vi "Send Core.vi"(6 "Severity Code (info)":T1=enum."info", 8 "Error In":errorcluster, 9 "Message Content":string, 10 "Message Tag":string, 11 "CS++DSCMsgLogger in":refnum<class "CS++DSCMsgLogger.lvclass">) -> (0 "Error Out":errorcluster, 3 "CS++DSCMsgLogger out":refnum<class "CS++DSCMsgLogger.lvclass">)   [LabVIEW 2014, in "CS++DSCMsgLogger.lvlib" / "CS++DSCMsgLogger.lvclass"]
doc: "Send mesage to central message logger."
uses:
  CS++DSCMsgLogger.lvclass
  CSPP_Core/Libraries/Base/Severity.ctl
  CS++DSCMsgLogger.lvclass/CS++DSCMsgLogger.ctl
  <vilib>/Utility/error.llb/DialogType.ctl
  CSPP_Core/Libraries/Base/CS++Base.lvlib
  <vilib>/lvdsc/NI_DSC.lvlib
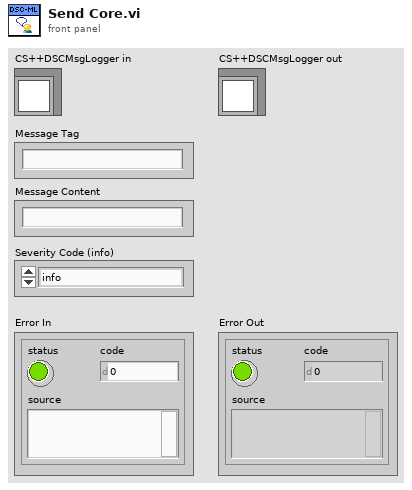
[diagram p1: front panel]
types:
  T1 = typedef "CS++Base.lvlib/Severity.ctl" = enum16{"emergency", "alert", "critical", "error", "warning", "notice", "info", "debug"}
  T2 = typedef "DialogType.ctl" = u16
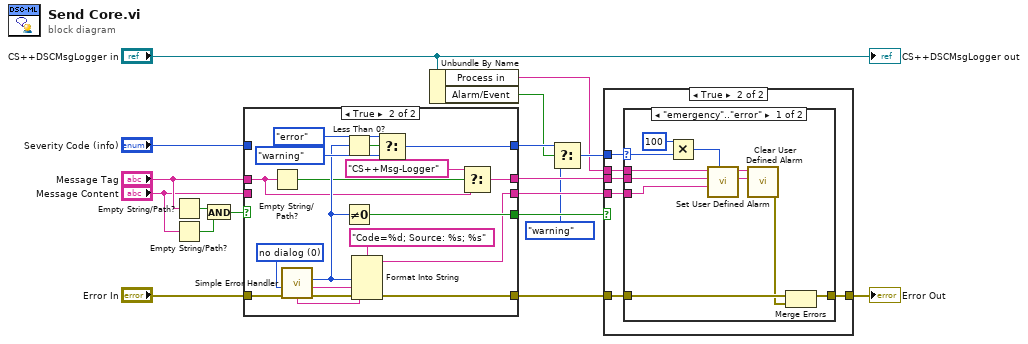
[diagram p0: block diagram]
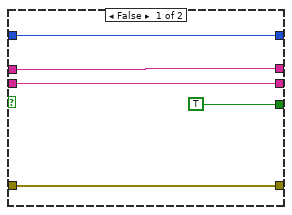
[diagram p2: hidden frame]
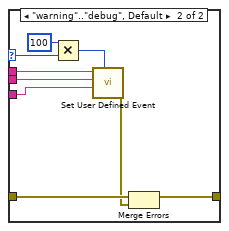
[diagram p4: hidden frame]
diagram:
  n1 = Empty String/Path?(string/path="Message Tag") -> (empty?=w12:bool)
  n2 = Empty String/Path?(string/path="Message Content") -> (empty?=w13:bool)
  n3 = And(x=w12, y=w13) -> (x .and. y?=w11:bool)
  n4 = case shown="True" w11 {
    tunnel: [w23 w36] -> w10
    tunnel: "Error In" -> [w23 w37]
    tunnel: [w22 w26] -> w9
    tunnel: "Message Tag" -> [w22 w24]
    tunnel: [w21 w29] -> w8
    tunnel: "Message Content" -> [w21 _]
    tunnel: [TRUE w40] -> w7
    tunnel: [w19 w38] -> w6
    tunnel: "Severity Code (info)" -> [w19 _]
    frame False {
    }
    frame True {
      w35 = T2 0 items=["no dialog", "OK message", "continue or stop message", "OK message + warnings", "continue/stop + warnings"] ("type of dialog (OK msg:1)")
      n5 = Empty String/Path?(string/path=w24) -> (empty?=w25:bool)
      n6 = call <vilib>:"Simple Error Handler.vi"("type of dialog (OK msg:1)"=w35, "error in (no error)"=w37) -> ("code out"=w33:i32, "source out"=w32:string, "error out"=w36:errorcluster, "message"=w31:string)  [unwired: 3 in, 1 out]
      n7 = Less Than 0?(x=w33) -> (x < 0?=w28:bool)
      n8 = Not Equal To 0?(x=w33) -> (x != 0?=w40:bool)
      n9 = Format Into String(format string="Code=%d; Source: %s; %s", w33, w32, w31) -> (resulting string=w29:string)  [unwired: 2 in, 1 out]
      n10 = Select(t=Severity."error" ("Severity Code (error)"), s=w28, f=Severity."warning" ("Severity Code (error)")) -> (s? t:f=w38:T1)
      n11 = Select(t="CS++Msg-Logger" ("Message Tag"), s=w25, f=w24) -> (s? t:f=w26:string)
    }
  }
  n12 = Unbundle By Name("CS++DSCMsgLogger in") -> ("Process in"=w2:string, "Alarm/Event"=w1:bool)
  n13 = Select(t=w6, s=w1, f=Severity."warning") -> (s? t:f=w5:T1)
  n14 = case shown="True" w7 {
    tunnel: w5 -> [_ w47]
    tunnel: w10 -> [w41 w46]
    tunnel: [w41 w45] -> w14
    tunnel: w9 -> [_ w44]
    tunnel: w8 -> [_ w43]
    tunnel: w2 -> [_ w42]
    frame False {
    }
    frame True {
      n15 = case shown="\"emergency\"..\"error\"" w47 {
        selector: w47 -> [w49 w62]
        tunnel: w44 -> [w52 w65]
        tunnel: w43 -> [w54 w64]
        tunnel: w46 -> [w55 w63]
        tunnel: [w56 w61] -> w45
        tunnel: w42 -> [w53 w60]
        frame "emergency".."error" {
          n16 = Multiply(x=100, y=w49) -> (x*y=w48:i32)
          n17 = call <vilib>:"Set User Defined Alarm.vi"("priority"=w48, "description"=w54, "alarm name"=w52, "process name"=w53) -> ()  [unwired: 7 in, 1 out]
          n18 = call <vilib>:"Clear User Defined Alarm.vi"("alarm name"=w52, "process name"=w53) -> ("error out"=w51:errorcluster)  [unwired: 9 in]
          n19 = Merge Errors(w55, w51) -> (w56:errorcluster)
        }
        frame "warning".."debug", Default {
          n20 = Multiply(x=100, y=w62) -> (x*y=w58:i32)
          n21 = call <vilib>:"Set User Defined Event.vi"("priority"=w58, "description"=w64, "event name"=w65, "process name"=w60) -> ("error out"=w59:errorcluster)  [unwired: 7 in]
          n22 = Merge Errors(w63, w59) -> (w61:errorcluster)
        }
      }
    }
  }
  "Error Out" <- w14
  "CS++DSCMsgLogger out" <- "CS++DSCMsgLogger in"
